vi "rotate XY graf test.vi"() -> ()   [LabVIEW 2019]
panel:
  out "Array":dbl[](array[numeric])
  in  "y":dbl=1.0 format="%#_13g"
  out "XY Graph":cluster{timestamp[], dbl[]}[](graph)
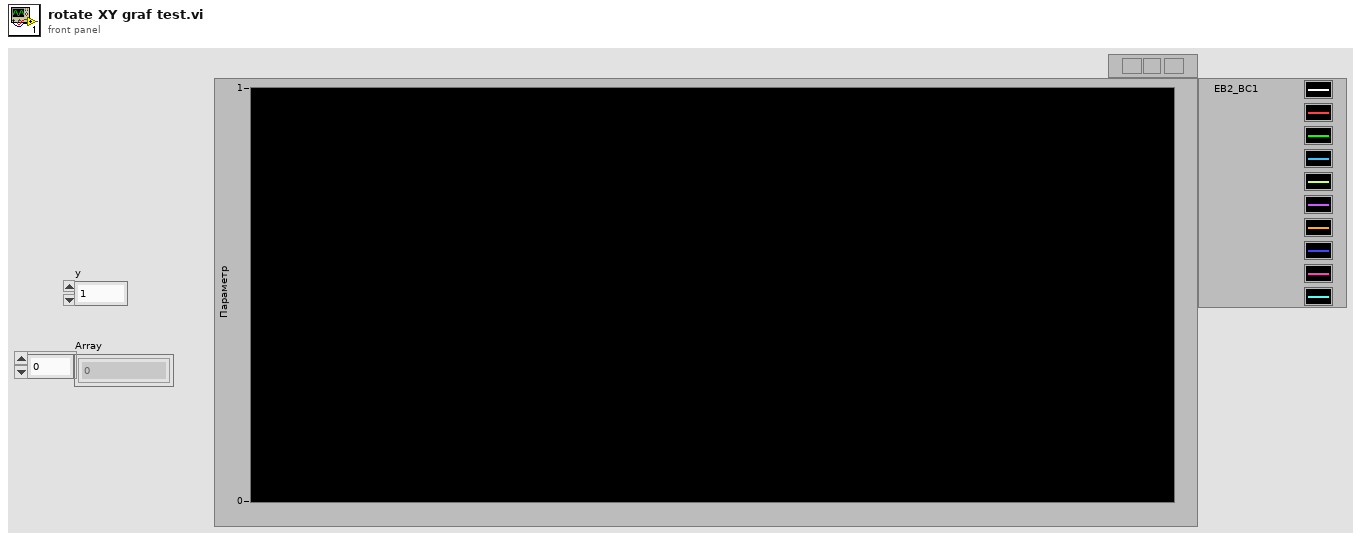
[diagram p1: front panel]
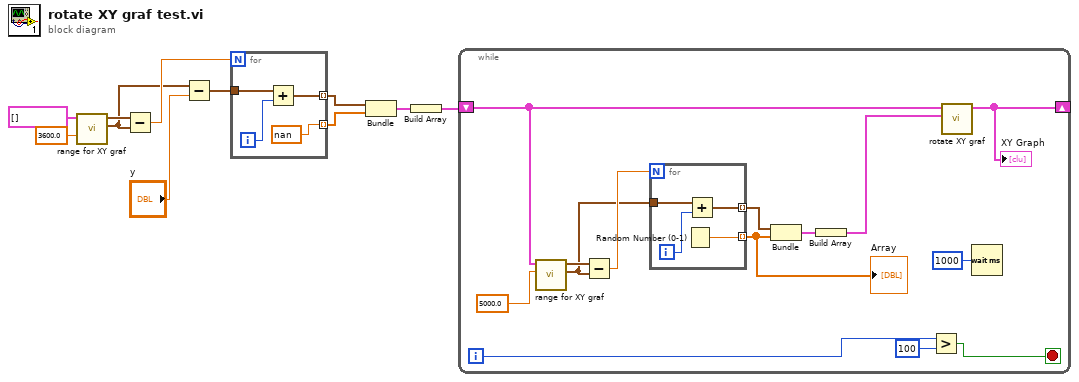
[diagram p0: block diagram]
diagram:
  n1 = call "range for XY graf.vi"("range"=3600.0, "XY Graf"=cluster{timestamp[], dbl[]}[] []) -> ("start time"=w2:timestamp, "end time"=w7:timestamp)  [unwired: 8 in]
  n2 = Subtract(x=w7, y=w2) -> (x-y=w3:dbl)
  n3 = Subtract(x=w2, y="y") -> (x-y=w1:timestamp)
  n4 = for {
    N: w3 -> [_]
    tunnel: w1 -> [w15]
    tunnel: [w13] -> w10 mode=indexing
    tunnel: [nan ("number (0 to 1)")] -> w9 mode=indexing
    i -> [w14]
    n5 = Add(x=w15, y=w14) -> (x+y=w13:timestamp)
  }
  n6 = Bundle(w10, w9) -> (w11:cluster{timestamp[], dbl[]})  [unwired: 1 in]
  n7 = Build Array(w11) -> (w8:cluster{timestamp[], dbl[]}[])
  n8 = while {
    shift-right: [w20] -> _
    shift-left: w8 -> [w29]
    i -> [w19]
    stop <- w17 stop-if-true
    n9 = call "range for XY graf.vi"("range"=5000.0, "XY Graf"=w29) -> ("start time"=w25:timestamp, "end time"=w27:timestamp)  [unwired: 8 in]
    n10 = Subtract(x=w27, y=w25) -> (x-y=w26:dbl)
    n11 = for {
      N: w26 -> [_]
      tunnel: w25 -> [w33]
      tunnel: [w31] -> w24 mode=indexing
      tunnel: [w30] -> w23 mode=indexing
      i -> [w32]
      n12 = Random Number (0-1)() -> (number: 0 to 1=w30:dbl)
      n13 = Add(x=w33, y=w32) -> (x+y=w31:timestamp)
    }
    "Array" <- w23
    n14 = Bundle(w24, w23) -> (w22:cluster{timestamp[], dbl[]})  [unwired: 1 in]
    n15 = Build Array(w22) -> (w21:cluster{timestamp[], dbl[]}[])
    n16 = Greater?(x=w19, y=100) -> (0:w17:bool)
    n17 = call "rotate XY graf.vi"("replased"=w21, "XY Graf in"=w29) -> ("XY Graf out"=w20:cluster{timestamp[], dbl[]}[])  [unwired: 9 in]
    "XY Graph" <- w20
    n18 = Wait (ms)(milliseconds to wait=u32 1000) -> ()  [unwired: 1 out]
  }
